vi "Get Lockin data module.vi"(8 "error in (no error)":errorcluster, 9 "Lockin address 1":string, 10 "Output data in":dbl[](array[numeric]), 11 "Lockin 1":bool) -> (0 "error out":errorcluster, 1 "Output data out":dbl[](array[numeric]), 2 "X mV":dbl, 3 "Y mV":dbl)   [LabVIEW 2024]
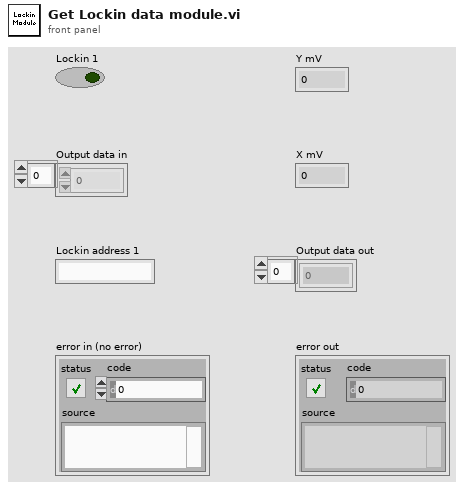
[diagram p1: front panel]
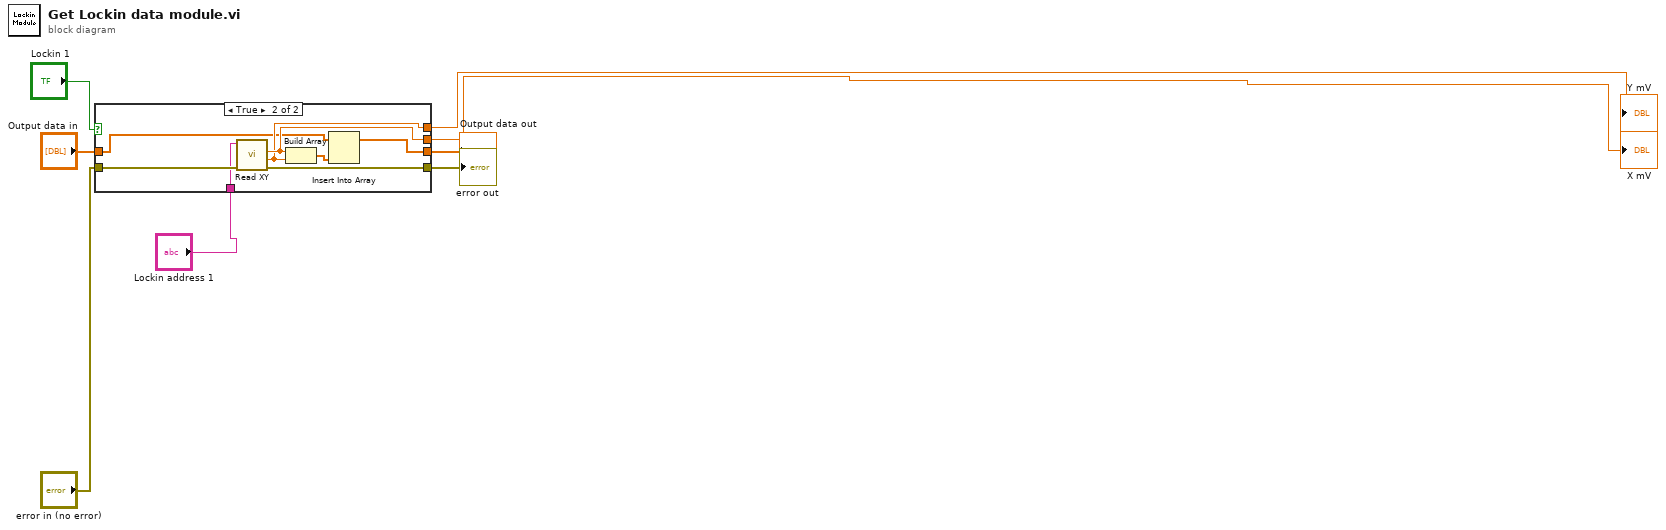
[diagram p0: block diagram]
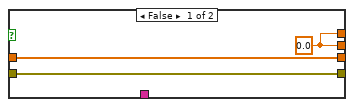
[diagram p2: hidden frame]
diagram:
  n1 = case shown="True" "Lockin 1" {
    tunnel: [w9 w18] -> w2
    tunnel: [w10 w19] -> w1
    tunnel: [w11 w16] -> w6
    tunnel: [w11 w15] -> w7
    tunnel: "error in (no error)" -> [w9 w14]
    tunnel: "Output data in" -> [w10 w13]
    tunnel: "Lockin address 1" -> [_ w12]
    frame False {
      w11 = 0.0 ("Y mV")
    }
    frame True {
      n2 = call "Read XY.vi"("error in (no error)"=w14, "VISA resource name"=w12) -> ("error out"=w18:errorcluster, "Y mV"=w15:dbl, "X mV"=w16:dbl)  [unwired: 5 in, 2 out]
      n3 = Build Array(w16, w15) -> (w17:dbl[])
      n4 = Insert Into Array(array=w13, new element=w17) -> (w19:dbl[])  [unwired: 1 in]
    }
  }
  "Y mV" <- w7
  "X mV" <- w6
  "error out" <- w2
  "Output data out" <- w1
